vi "LVClass_WavefrontCorrector ctor Instance.vi"(0 "WavefrontCorrector (const)":refnum<class "WavefrontCorrector.lvclass">, 5 "PathToWavefrontCorrectorSetupFile":path, 11 "error in (no error)":errorcluster) -> (4 "WavefrontCorrector (new)":refnum<class "WavefrontCorrector.lvclass">, 15 "error out":errorcluster)   [LabVIEW 2020, in "WavefrontCorrector.lvclass"]
doc: "WavefrontCorrector constructor.\n\n--------------------------------------------------------------------------------\n\n<B>correctorIn </B> : Constant Pointer to WavefrontCorrector object.\n<B>correctorOut </B> : Constant Pointer to WavefrontCorrector object.\n<B>config_file_path </B> : Absolute path to Wavefront corrector configuration file.\n<B>ErrorIn </B> : Error\n<B>ErrorOut </B> : Error\n\n--------------------------------------------------------------------------------"
uses:
  WavefrontCorrector.lvclass
  WavefrontCorrectorSet.lvclass
  Wavefront Corrector states - ONE.ctl
  WavefrontCorrector.lvclass/WavefrontCorrector.ctl
  Handle creation.ctl
  LVClass_WavefrontCorrectorSet Read AllWavefrontCorrectorParametersProperties.vi
  LVClass_WavefrontCorrectorSet Read AllValueSetAndGet.vi
  LVClass_WavefrontCorrectorSet Read AllValueGet.vi
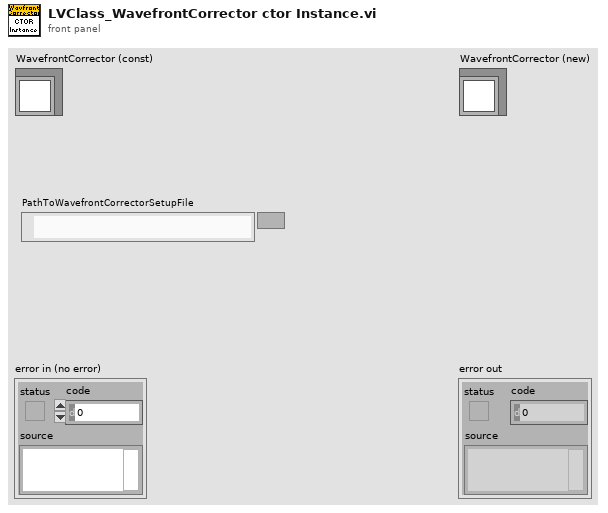
[diagram p1: front panel]
types:
  T1 = typedef "Wavefront Corrector states - ONE.ctl" = cluster{"Max":sgl, "Min":sgl, "Validity":enum16{"valid", "fixed", "invalid"}, "Fixed_Position":sgl}
  T2 = typedef "Handle creation.ctl" = enum16{"By ctor", "By write function"}
  T3 = typedef "WavefrontCorrectorSpecifications.ctl" = cluster{"Mirror name":string, "Plugin name":string, "Serial number":string, "Revision":string, "Number of commands":i32, "Sleep after command apply (ms)":i32, "Has internal memory ?":bool}
  T4 = typedef "ParameterID.ctl" = cluster{"Name":string, "ConnectionParameter?":bool, "Type":T5, "Authorization":T6, "OnFlyAuthorization":T7, "StringValue":string, "Value":dbl, "Min":dbl, "Max":dbl, "BooleanValue":bool, "StringParameterList":string[]}
  T5 = typedef "CameraParameters_Type.ctl" = enum16{"Integer", "Real", "String", "Boolean"}
  T6 = typedef "CameraParameters_Authorization.ctl" = enum16{"Disable", "Gettable", "Settable - Gettable"}
  T7 = typedef "CameraParameters_OnFlyAuthorization.ctl" = enum16{"None", "Gettable", "Settable", "Settable - Gettable"}
  T8 = typedef "CameraParametersSetup.ctl" = cluster{"Name":string, "Type":T5, "Value":dbl, "BooleanValue":bool, "StringValue":string, "ConnectionParameter":bool}
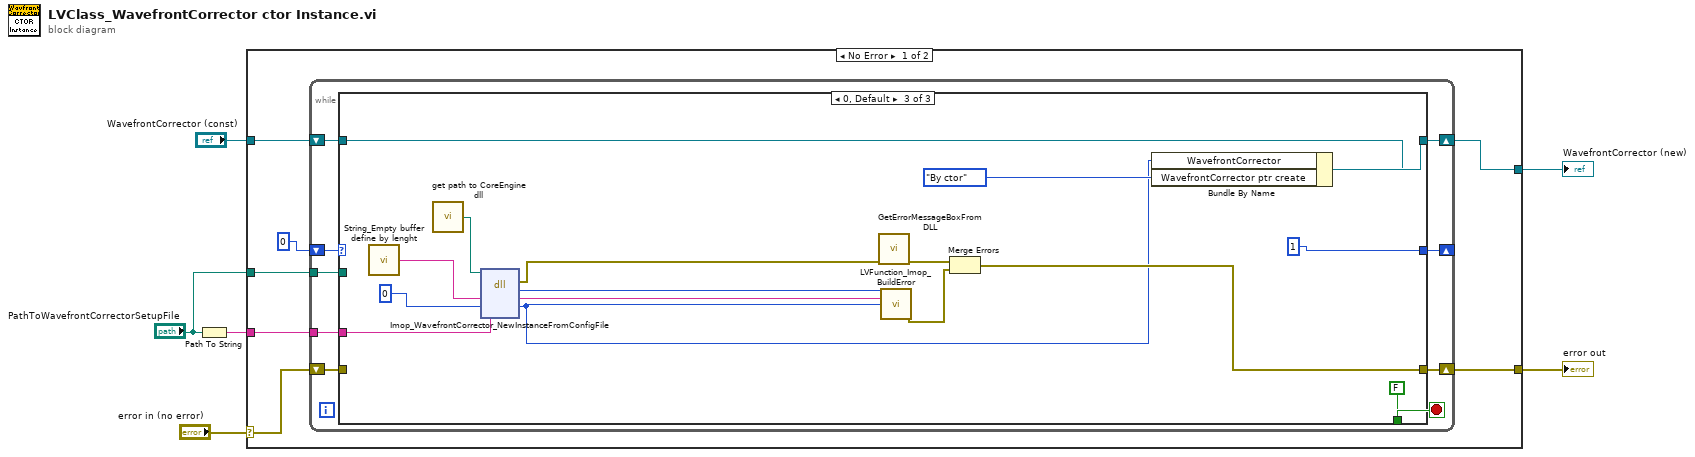
[diagram p0: block diagram]
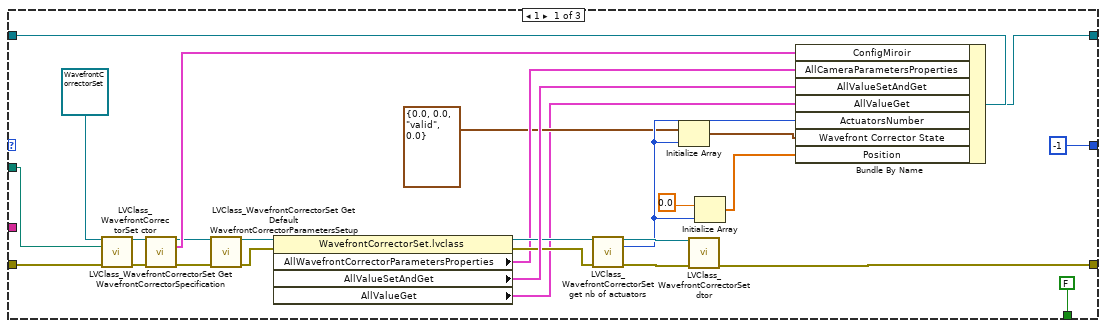
[diagram p2: hidden frame]
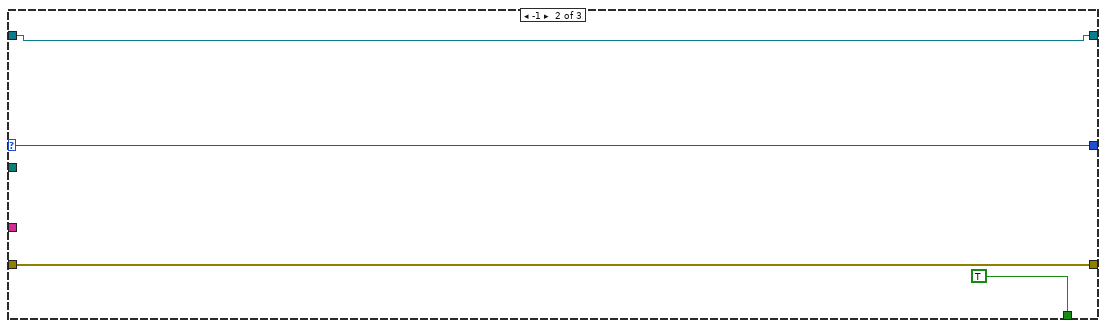
[diagram p3: hidden frame]
diagram:
  n1 = Path To String(path="PathToWavefrontCorrectorSetupFile") -> (string=w6:string)
  n2 = case shown="No Error" "error in (no error)" {
    selector: "error in (no error)" -> [w8 w71]
    tunnel: [w7 w71] -> w3
    tunnel: [w12 w70] -> w2
    tunnel: "WavefrontCorrector (const)" -> [w13 w70]
    tunnel: w6 -> [w11 _]
    tunnel: "PathToWavefrontCorrectorSetupFile" -> [w9 _]
    frame No Error {
      n3 = while {
        tunnel: w11 -> [w21]
        shift-right: [w19] -> _
        shift-left: 0 -> [w20]
        tunnel: w9 -> [w18]
        shift-right: [w15] -> w7
        shift-left: w8 -> [w16]
        shift-right: [w22] -> w12
        shift-left: w13 -> [w17]
        stop <- w14 stop-if-true
        n4 = case shown="0, Default" w20 {
          selector: w20 -> [_ w53 _]
          tunnel: [w37 w50 w62] -> w22
          tunnel: [w38 w52 w59] -> w15
          tunnel: w21 -> [_ _ w58]
          tunnel: [-1 w53 1] -> w19
          tunnel: w18 -> [w47 _ _]
          tunnel: w17 -> [w46 w50 w55]
          tunnel: w16 -> [w43 w52 _]
          tunnel: [FALSE TRUE FALSE] -> w14
          frame 1 {
            n5 = call "LVClass_WavefrontCorrectorSet ctor.vi"("WavefrontCorrectorSet (const)"=refnum<class "WavefrontCorrectorSet.lvclass"> refnum ("WavefrontCorrectorSet.lvclass"), "PathToWavefrontCorrectorSetupFile"=w47, "error in (no error)"=w43) -> ("WavefrontCorrectorSet (new)"=w49:refnum<class "WavefrontCorrectorSet.lvclass">, "error out"=w44:errorcluster)  [unwired: 11 in]
            n6 = call "LVClass_WavefrontCorrectorSet Get WavefrontCorrectorSpecification.vi"("WavefrontCorrectorSet in"=w49, "error in (no error)"=w44) -> ("WavefrontCorrectorSet out"=w31:refnum<class "WavefrontCorrectorSet.lvclass">, "ConfigMiroir"=w45:T3, "error out"=w32:errorcluster)  [unwired: 11 in]
            n7 = call "LVClass_WavefrontCorrectorSet Get Default WavefrontCorrectorParametersSetup.vi"("WavefrontCorrectorSet in"=w31, "error in (no error)"=w32) -> ("WavefrontCorrectorSet out"=w29:refnum<class "WavefrontCorrectorSet.lvclass">, "error out"=w27:errorcluster)  [unwired: 9 in, 3 out]
            n8 = property class="WavefrontCorrectorSet.lvclass"(reference=w29, error in=w27) -> (reference out=w28:refnum<class "WavefrontCorrectorSet.lvclass">, error out=w26:errorcluster, "AllWavefrontCorrectorParametersProperties"=w25:T4[], "AllValueSetAndGet"=w30:T8[], "AllValueGet"=w23:T8[])
            n9 = call "LVClass_WavefrontCorrectorSet get nb of actuators.vi"("WavefrontCorrectorSet in"=w28, "error in (no error)"=w26) -> ("WavefrontCorrectorSet out"=w40:refnum<class "WavefrontCorrectorSet.lvclass">, "ActuatorsNumber"=w34:i32, "error out"=w39:errorcluster)  [unwired: 11 in]
            n10 = Initialize Array(T1 {"Max"=0.0, "Min"=0.0, "Validity"=enum."valid", "Fixed_Position"=0.0} ("Actuator State"), w34) -> (w36:T1[])
            n11 = call "LVClass_WavefrontCorrectorSet dtor.vi"("WavefrontCorrectorSet in"=w40, "error in (no error)"=w39) -> ("error out"=w38:errorcluster)  [unwired: 12 in, 1 out]
            n12 = Initialize Array(sgl 0.0 ("Numeric"), w34) -> (w33:sgl[])
            n13 = Bundle By Name(cluster=w46, "ConfigMiroir"=w45, "AllCameraParametersProperties"=w25, "AllValueSetAndGet"=w30, "AllValueGet"=w23, "ActuatorsNumber"=w34, "Wavefront Corrector State"=w36, "Position"=w33) -> (w37:refnum<class "WavefrontCorrector.lvclass">)
          }
          frame -1 {
          }
          frame 0, Default {
            n14 = call "String_Empty buffer define by lenght.vi"() -> ("Empty buffer"=w69:string)  [unwired: 1 in]
            n15 = call "get path to CoreEngine dll.vi"() -> ("path to wavekit library"=w66:path)  [unwired: 14 in, 1 out]
            n16 = dll-call lib="D:/soft/HASO_v3/SVN_trunk/ImOpCoreEngine4_LV2011/DLLs/c_interface_vc100.dll" fn="Imop_WavefrontCorrector_NewInstanceFromConfigFile"(path in=w66, "message"=w69, "WavefrontCorrector"=0 ("Pupil"), "Config_file_path"=w58) -> (error out=w65:errorcluster, "return type"=w67:i32, "message"=w68:string, "WavefrontCorrector"=w54:i64)  [unwired: 3 in, 1 out]
            n17 = call "GetErrorMessageBoxFromDLL.vi"("error IN"=w65) -> ("error OUT"=w61:errorcluster)  [unwired: 10 in]
            n18 = call "LVFunction_Imop_BuildError.vi"("code"=w67, "String to Prepend to source (\"\")"=w68, "Adresse"=w54) -> ("error out"=w60:errorcluster)  [unwired: 12 in]
            n19 = Merge Errors(w61, w60) -> (w59:errorcluster)
            n20 = Bundle By Name(cluster=w55, "WavefrontCorrector"=w54, "WavefrontCorrector ptr create"=Handle_creation."By ctor" ("Pupil ptr create")) -> (w62:refnum<class "WavefrontCorrector.lvclass">)
          }
        }
      }
    }
    frame Error {
    }
  }
  "error out" <- w3
  "WavefrontCorrector (new)" <- w2
